vi "Temperature Limit.vi"() -> ()   [LabVIEW 2012]
doc: "This VI simulates the acquisition of temperature, graphs the temperature, and notifies the user if the temperature is over the limit."
uses:
  <vilib>/ErrorRing/Error Ring.xnode
panel:
  in  "Start":bool
  in  "Delta t (ms)":i32(slide)=400 scale=50.0..500.0
  in  "Stop":bool
  in  "High Limit":dbl=28.0 format="%.2f"
  out "Temperature":cluster{"Temperature":dbl, "High Limit":dbl}(graph)={"Temperature"=85.88749999999999, "High Limit"=80.0}
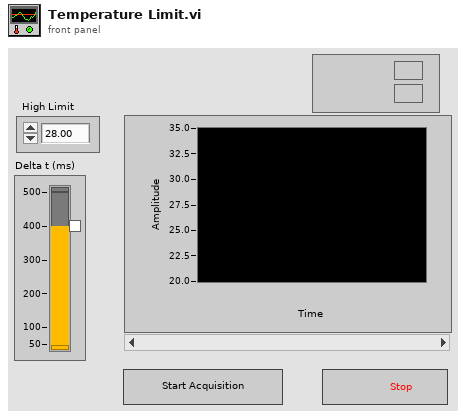
[diagram p1: front panel]
types:
  T1 = enum16{"Always On", "Always Off", "Off While Running"}
  T2 = cluster{"Temperature Value":dbl, "High Limit":dbl}
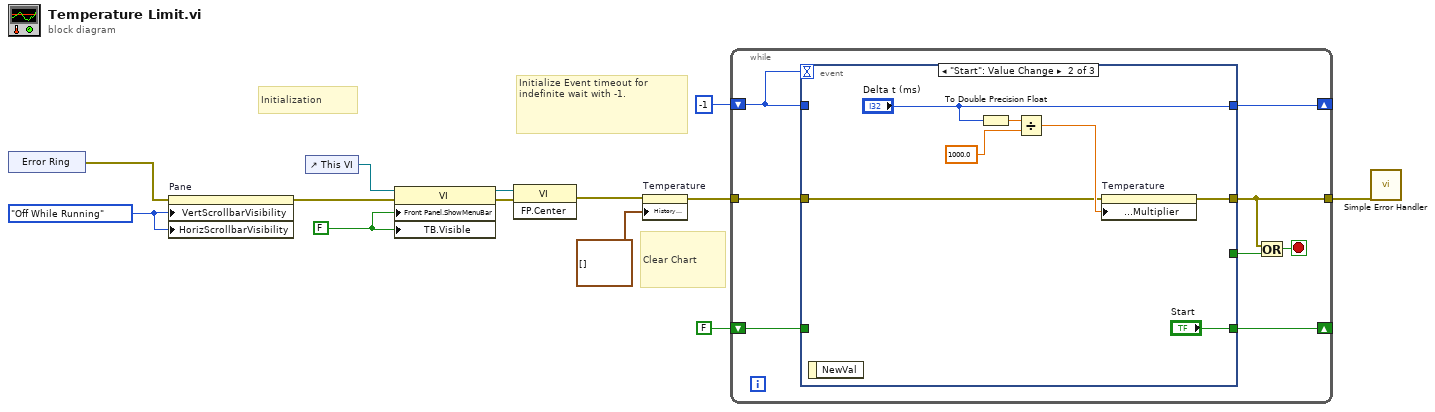
[diagram p0: block diagram]
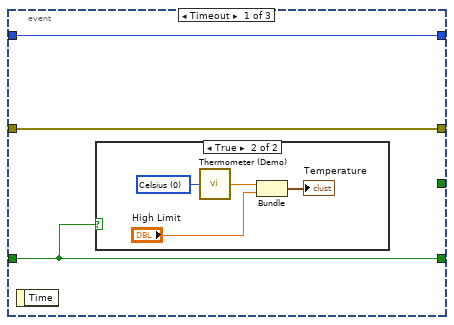
[diagram p2: hidden frame]
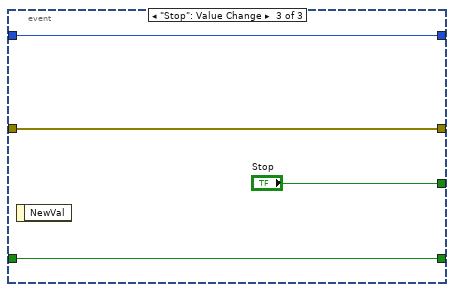
[diagram p4: hidden frame]
diagram:
  w3 = T1."Off While Running" ("Horizontal Scrollbar Visibility")
  w8 = FALSE
  # "Clear Chart"
  # "Initialize Event timeout for indefinite wait with -1."
  # "Initialization"
  n1 = xnode "Error Ring"() -> ("error out"=w1:errorcluster)
  n2 = property on="Pane" class="Pane"(error in=w1, "VertScrollbarVisibility"=w3, "HorizScrollbarVisibility"=w3) -> (error out=w4:errorcluster)  [unwired: 1 in, 1 out]
  n3 = control-ref of="This VI"() -> (w5:refnum<vi>)
  n4 = property class="VI"(reference=w5, error in=w4, "Front Panel.ShowMenuBar"=w8, "TB.Visible"=w8) -> (reference out=w7:refnum<vi>, error out=w6:errorcluster)
  n5 = invoke class="VI" method="FP.Center"(reference=w7, error in=w6) -> (error out=w2:errorcluster)  [unwired: 1 in, 2 out]
  n6 = property on="Temperature" class="WFChart (strict)"(error in=w2, "History Data"=cluster{"Temperature":dbl, "High Limit":dbl}[] []) -> (error out=w12:errorcluster)  [unwired: 1 in, 1 out]
  n7 = while {
    tunnel: w12 -> [w21]
    tunnel: [w19] -> w10
    shift-right: [w17] -> _
    shift-left: FALSE ("Start") -> [w16]
    shift-right: [w15] -> _
    shift-left: -1 ("Delta t (ms)") -> [w14]
    stop <- w20 stop-if-true
    n8 = event shown="[1] \"Start\": Value Change" {
      selector: _ -> [_ _ _]
      dyn-events: _ -> [_ _ _]
      timeout: w14 -> [_ _ _]
      tunnel: [_ _ "Stop"] -> w18
      tunnel: w21 -> [w24 w29 w38]
      tunnel: [w24 w35 w38] -> w19
      tunnel: [w22 "Start" w37] -> w17
      tunnel: w16 -> [w22 _ w37]
      tunnel: [w23 "Delta t (ms)" w36] -> w15
      tunnel: w14 -> [w23 _ w36]
      event Timeout {
        n9 = event-data() -> ()  [unwired: 1 in, 1 out]
        n10 = case shown="True" w22 {
          frame False {
          }
          frame True {
            w25 = u16 0 items=["Celsius", "Fahrenheit"] ("Units (0: Celsius)")
            n11 = call "Thermometer (Demo).vi"("Units (0: Celsius)"=w25) -> ("Temperature Value"=w26:dbl)
            n12 = Bundle("Temperature Value"=w26, "High Limit"="High Limit") -> (→"Temperature":T2)  [unwired: 1 in]
          }
        }
      }
      event "Start": Value Change {
        n13 = event-data() -> ()  [unwired: 1 in, 1 out]
        n14 = To Double Precision Float(number="Delta t (ms)") -> (double precision float=w34:dbl)
        n15 = Divide(x=w34, y=1000.0) -> (x/y=w32:dbl)
        n16 = property on="Temperature" class="WFChart (strict)"(error in=w29, "X Scale.Offset and Multiplier:Multiplier"=w32) -> (error out=w35:errorcluster)  [unwired: 1 in, 1 out]
      }
      event "Stop": Value Change {
        n17 = event-data() -> ()  [unwired: 1 in, 1 out]
      }
    }
    n18 = Or(x=w19, y=w18) -> (x .or. y?=w20:bool)
  }
  n19 = call <vilib>:"Simple Error Handler.vi"("error in (no error)"=w10) -> ()  [unwired: 4 in, 5 out]
